vi "ICNC Move Profile Abs Buf.vi"(0 "Axis":u32, 1 "PositionZ":i32, 2 "PositionB":i32, 5 "Speed":u32, 7 "PositionX":i32, 9 "PositionY":i32, 11 "error in (no error)":errorcluster caption="entrée d'erreur (pas d'erreur)", 12 "PositionA":i32, 13 "BufferRequired":u32) -> (4 "BufferRequired out":u32, 6 "function return":u32, 15 "error out":errorcluster caption="sortie d'erreur")   [LabVIEW 2012, in "ICNC2.lvlib"]
doc: "DWORD ICNC_MoveProfileAbsBuf ( DWORD Axis,\n DWORD Speed,\n INT PositionX,\n INT PositionY,\n INT PositionZ,\n INT PositionA,\n INT PositionB,\n DWORD *BufferRequired=NULL);"
uses:
  <userlib>/ICNC/ICNC2.lvlib
  <userlib>/ICNC/ICNC2.dll
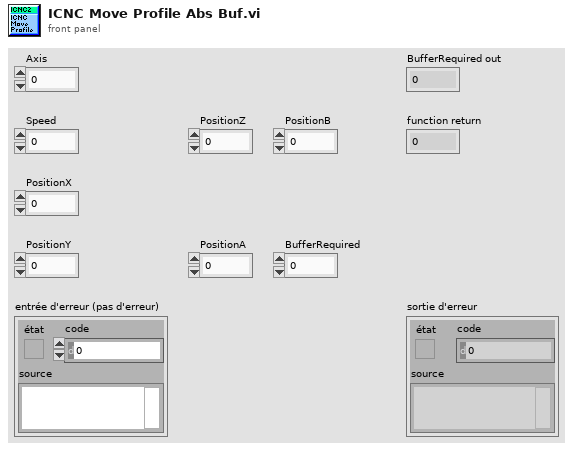
[diagram p1: front panel]
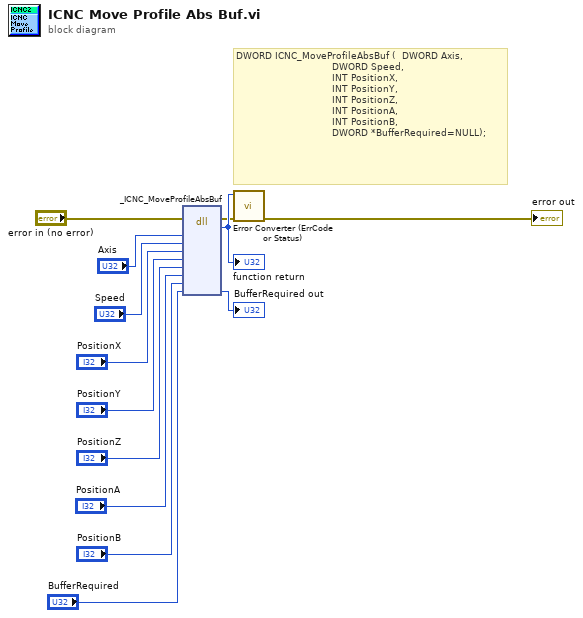
[diagram p0: block diagram]
diagram:
  # "DWORD ICNC_MoveProfileAbsBuf (  DWORD Axis,\n                                DWORD Speed,\n                                INT PositionX,\n                                INT PositionY,\n                                INT PositionZ,\n                                INT PositionA,\n                                INT PositionB,\n                                DWORD *BufferRequired=NULL);"
  n1 = dll-call lib="C:/Program Files (x86)/National Instruments/LabVIEW 2012/user.lib/ICNC/ICNC2.*" fn="_ICNC_MoveProfileAbsBuf"(error in="error in (no error)", "Axis"="Axis", "Speed"="Speed", "PositionX"="PositionX", "PositionY"="PositionY", "PositionZ"="PositionZ", "PositionA"="PositionA", "PositionB"="PositionB", "BufferRequired"="BufferRequired") -> (error out=w2:errorcluster, w13:u32, "BufferRequired"=→"BufferRequired out":u32)  [unwired: 9 in, 1 out]
  "function return" <- w13
  n2 = call <userlib>:"Error Converter (ErrCode or Status).vi"("error in (no error)"=w2, "error code"=w13) -> ("error out"=→"error out":errorcluster)  [unwired: 9 in]
